vi "Measure_dC_dV.vi"(5 "Junction Name":string, 6 "UiDefinition":T1, 7 ".NET Refnum":refnum<k24>, 8 "new file path (Not A Path if cancelled)":path, 10 "appended path":path, 11 ".NET Refnum in":refnum<k24>) -> (0 "error out":errorcluster, 3 "Cluster":cluster{dbl[], dbl[]})   [LabVIEW 2020]
uses:
  UIReferences.ctl
  C:/Users/User/Desktop/Automation/CurrentVersion/LabviewDXFViewer/bin/Release/LabviewDXFViewer.exe
  LabviewDXFViewer/bin/Release/LabviewDXFViewer.exe
  <vilib>/Analysis/6fits.llb/Curve Fitting Criteria.ctl
  <vilib>/Utility/file.llb/Write Delimited Spreadsheet (string).vi
  <vilib>/Utility/file.llb/Write Delimited Spreadsheet (DBL).vi
  <vilib>/Analysis/NI_AALPro.lvlib
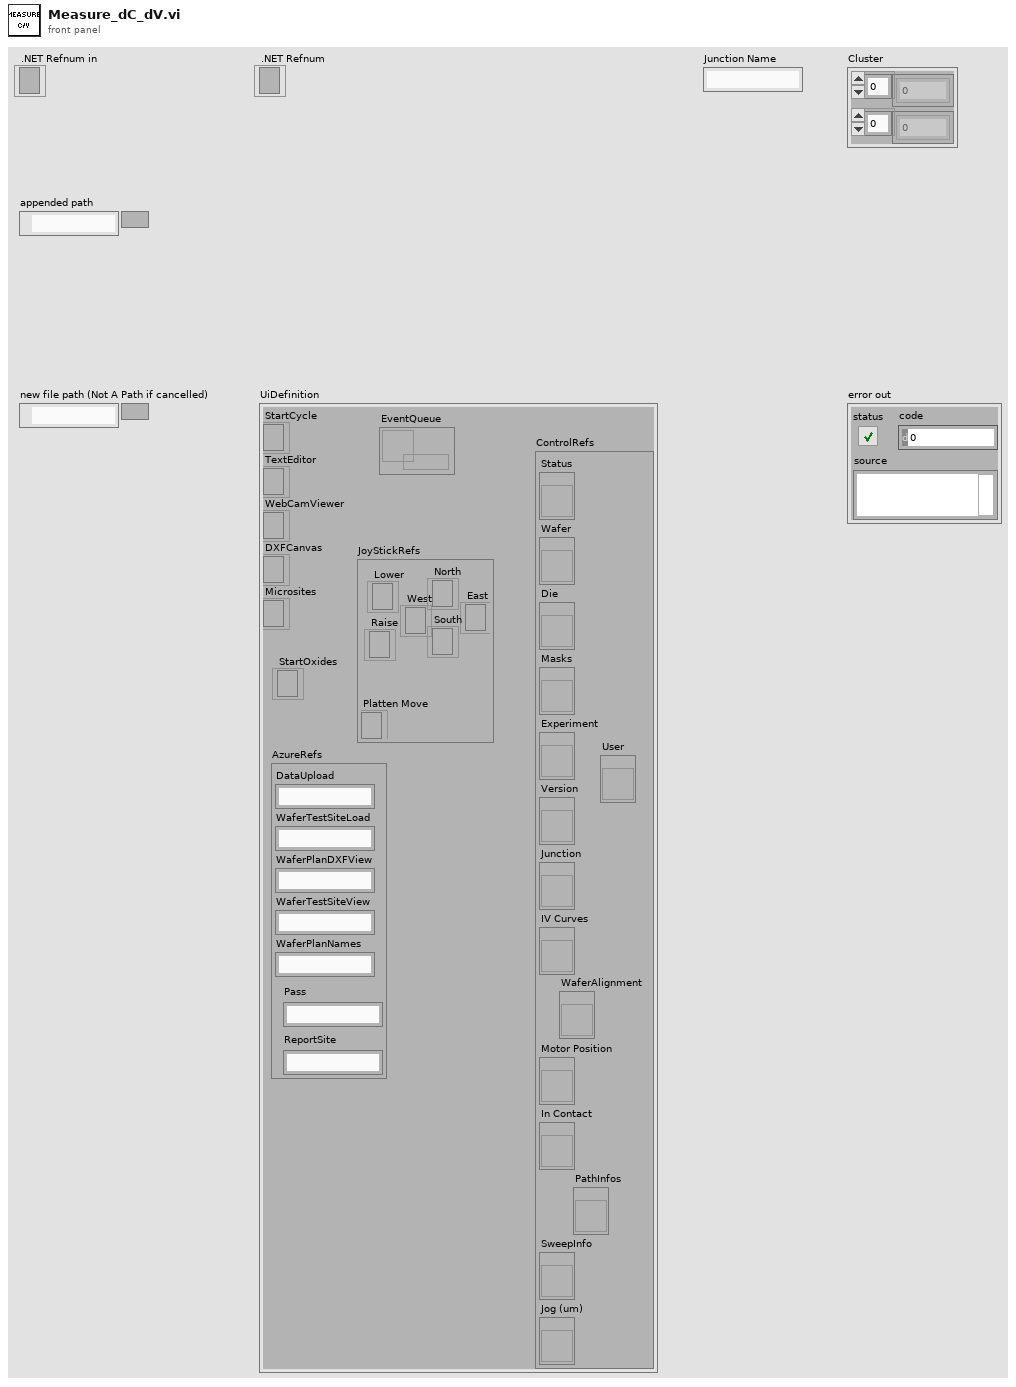
[diagram p1: front panel]
types:
  T1 = typedef "UIReferences.ctl" = cluster{"StartCycle":refnum<k24>, "TextEditor":refnum<k24>, "WebCamViewer":refnum<k24>, "DXFCanvas":refnum<k24>, "Microsites":refnum<k24>, "JoyStickRefs":cluster{"North":refnum<k24>, "Lower":refnum<k24>, "Raise":refnum<k24>, "Platten Move":refnum<k24>, "West":refnum<k24>, "East":refnum<k24>, "South":refnum<k24>}, "AzureRefs":cluster{"DataUpload":string, "WaferTestSiteLoad":string, "WaferPlanDXFView":string, "WaferTestSiteView":string, "WaferPlanNames":string, "Pass":string, "ReportSite":string}, "ControlRefs":cluster{"Status":refnum<vi>, "Wafer":refnum<vi>, "Die":refnum<vi>, "Masks":refnum<vi>, "Experiment":refnum<vi>, "Version":refnum<vi>, "Junction":refnum<vi>, "IV Curves":refnum<vi>, "Motor Position":refnum<vi>, "In Contact":refnum<vi>, "SweepInfo":refnum<vi>, "Jog (um)":refnum<vi>, "PathInfos":refnum<vi>, "User":refnum<vi>, "WaferAlignment":refnum<vi>}, "EventQueue":refnum<queue>, "StartOxides":refnum<k24>}
  T2 = typedef "NI_AALPro.lvlib/Curve Fitting Criteria.ctl" = u16
  T3 = typedef "CapacitanceInfos.ctl" = cluster{"Conductance":dbl, "CapacitanceIV":dbl, "Intercept":dbl, "CapacitanceSW":dbl, "Sum":dbl, "CapacitanceInfos":T4[], "CapacitancePhase":dbl, "dC/dV":dbl}
  T4 = typedef "CapacitanceRecord.ctl" = cluster{"Freq":dbl, "Vpp":dbl, "PhaseS":dbl, "Irms":dbl, "PhaseC":dbl, "Theta":dbl, "VDrive":dbl, "Capacitance":dbl, "Other":dbl}
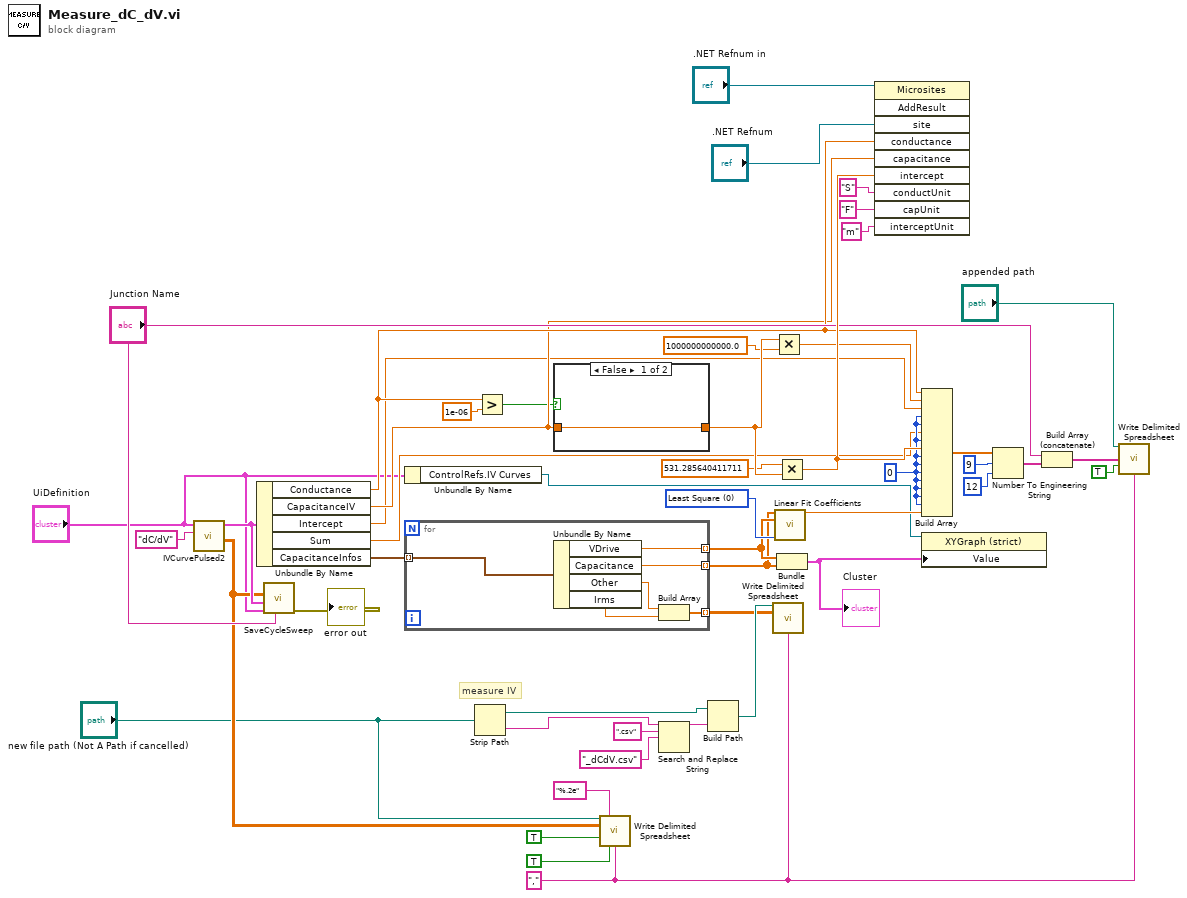
[diagram p0: block diagram]
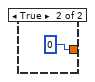
[diagram p2: hidden frame]
diagram:
  w2 = "," ("delimiter (\\t)")
  w45 = T2 0 items=["Least Square", "Least Absolute Residual", "Bisquare"] ("method")
  w42 = 0
  # "measure IV"
  n1 = call "IVCurvePulsed2.vi"("Program"="dC/dV", "UiDefinition"="UiDefinition") -> ("appended array"=w21:dbl[][], "InfoCluster"=w34:T3)  [unwired: 8 in]
  n2 = Unbundle By Name(w34) -> ("Conductance"=w36:dbl, "CapacitanceIV"=w35:dbl, "Intercept"=w24:dbl, "Sum"=w25:dbl, "CapacitanceInfos"=w37:T4[])
  n3 = call "SaveCycleSweep.vi"("JunctionName"="Junction Name", "UiDefinition 2"="UiDefinition", "InfoCluster"=w34, "appended array"=w21) -> ("error out"=→"error out":errorcluster)  [unwired: 7 in]
  n4 = Unbundle By Name("UiDefinition") -> ("ControlRefs.IV Curves"=w7:refnum<vi>)
  n5 = for {
    tunnel: w37 -> [w55] mode=indexing
    tunnel: [w54] -> w44 mode=indexing
    tunnel: [w53] -> w43 mode=indexing
    tunnel: [w52] -> w1 mode=indexing
    n6 = Unbundle By Name(w55) -> ("VDrive"=w54:dbl, "Capacitance"=w53:dbl, "Other"=w51:dbl, "Irms"=w50:dbl)
    n7 = Build Array(w51, w50) -> (w52:dbl[])
  }
  n8 = Strip Path(path="new file path (Not A Path if cancelled)") -> (stripped path=w8:path, name=w12:string)
  n9 = Greater?(x=w36, y=1e-06) -> (0:w28:bool)
  n10 = case shown="False" w28 {
    tunnel: [w56 0] -> w48
    tunnel: w35 -> [w56 _]
    frame False {
    }
    frame True {
    }
  }
  n11 = call-poly <vilib>:"Write Delimited Spreadsheet.vi"("file path (dialog if empty)"="new file path (Not A Path if cancelled)", "format (%.3f)"="%.2e", "2D data"=w21, "append to file? (new file:F)"=TRUE, "transpose? (no:F)"=TRUE, "delimiter (\\t)"=w2) -> ()  [unwired: 8 in, 2 out]
  n12 = Search and Replace String(input string=w12, search string=".csv", replace string="_dCdV.csv" ("replace string (\"\")")) -> (result string=w9:string)  [unwired: 5 in, 3 out]
  n13 = Build Path(base path=w8, name or relative path=w9) -> (appended path=w3:path)
  n14 = call-poly <vilib>:"Write Delimited Spreadsheet.vi"("file path (dialog if empty)"=w3, "2D data"=w1, "delimiter (\\t)"=w2) -> ()  [unwired: 11 in, 2 out]
  n15 = Multiply(x=w48, y=1000000000000.0) -> (x*y=w26:dbl)
  n16 = call <vilib>:"Linear Fit Coefficients.vi"("Y"=w43, "X"=w44, "method"=w45) -> ("slope"=w46:dbl)  [unwired: 10 in, 2 out]
  n17 = Multiply(x=531.285640411711, y=w48) -> (x*y=w49:dbl)
  n18 = Bundle(w44, w43) -> (w5:cluster{dbl[], dbl[]})  [unwired: 1 in]
  "Cluster" <- w5
  n19 = invoke class="Microsites" method="AddResult"(reference=".NET Refnum in", "site"=".NET Refnum", "conductance"=w36, "capacitance"=w35, "intercept"=w49, "conductUnit"="S", "capUnit"="F", "interceptUnit"="m") -> ()  [unwired: 2 in, 10 out]
  n20 = Build Array(w36, w26, w24, w42, w42, w25, w42, w49, w42, w42, w42, w42, w42, w42, w42, w46) -> (w23:dbl[])
  n21 = property class="XYGraph (strict)"(reference=w7, "Value"=w5) -> ()  [unwired: 1 in, 2 out]
  n22 = Number To Engineering String(2:i16 12 ("precision (6)"), 3:i16 9 ("width (-)"), 4:w23) -> (0:w15:string[])  [unwired: 1 in]
  n23 = Build Array (concatenate)("Junction Name", w15) -> (w17:string[])
  n24 = call-poly <vilib>:"Write Delimited Spreadsheet.vi"("file path (dialog if empty)"="appended path", "1D data"=w17, "append to file? (new file:F)"=TRUE, "delimiter (\\t)"=w2) -> ()  [unwired: 10 in, 2 out]
